vi "Write_GenericData.vi"(8 "error in (no error)":errorcluster, 10 "Data.CommandOrigin":T1, 11 "SubsystemData in":refnum<class "SubsystemData.lvclass">) -> (0 "error out":errorcluster, 3 "SubsystemData out":refnum<class "SubsystemData.lvclass">)   [LabVIEW 2017, in "SubsystemData.lvclass"]
uses:
  SubsystemData.lvclass
  CommandOrigin.ctl
  SubsystemData.lvclass/SubsystemData.ctl
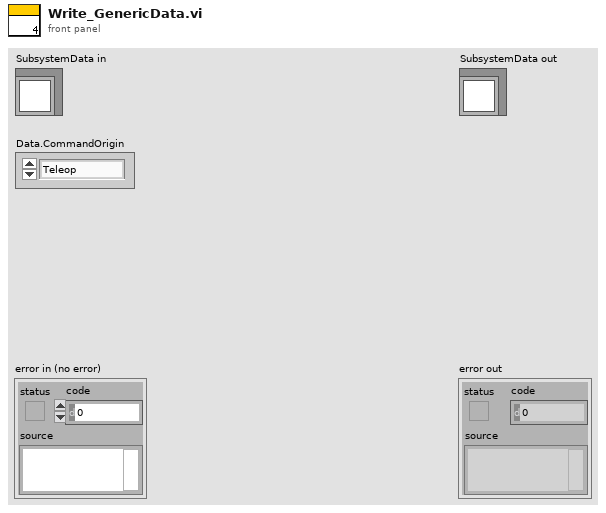
[diagram p1: front panel]
types:
  T1 = typedef "SubsystemData.lvclass/CommandOrigin.ctl" = enum16{"Teleop", "Auto"}
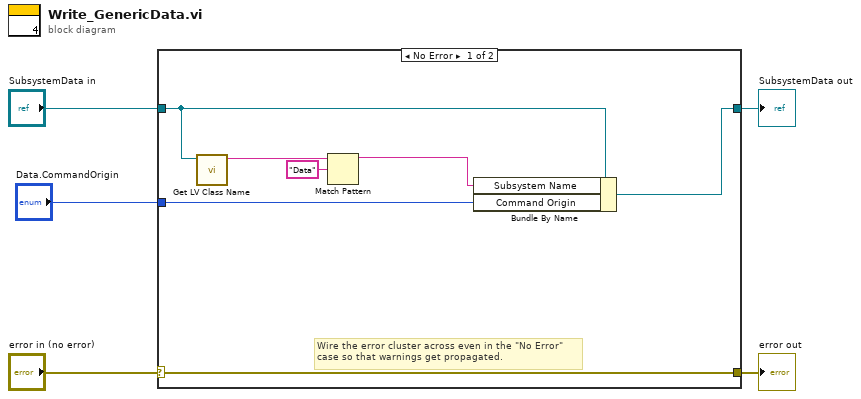
[diagram p0: block diagram]
diagram:
  n1 = case shown="No Error" "error in (no error)" {
    selector: "error in (no error)" -> [w12 w14]
    tunnel: [w12 w14] -> w4
    tunnel: [w7 w13] -> w2
    tunnel: "SubsystemData in" -> [w6 w13]
    tunnel: "Data.CommandOrigin" -> [w11 _]
    frame No Error {
      # "Wire the error cluster across even in the \"No Error\"\ncase so that warnings get propagated."
      n2 = call <vilib>:"Get LV Class Name.vi"("object"=w6) -> ("class name"=w10:string)  [unwired: 9 in, 1 out]
      n3 = Match Pattern(string=w10, regular expression="Data") -> (before substring=w8:string)  [unwired: 1 in, 3 out]
      n4 = Bundle By Name(cluster=w6, "Subsystem Name"=w8, "Command Origin"=w11) -> (w7:refnum<class "SubsystemData.lvclass">)
    }
    frame Error {
    }
  }
  "error out" <- w4
  "SubsystemData out" <- w2
